vi "Script.vi"(7 "_Rescript in":refnum<class "_Rescript.lvclass">, 8 "error in":errorcluster) -> (0 "error out":errorcluster, 5 "_Rescript out":refnum<class "_Rescript.lvclass">)   [LabVIEW 2025, in "_Rescript.lvlib" / "Msg.lvlib"]
uses:
  Msg.lvlib
  _Rescript/_Rescript.lvclass
  _Shared/Name Specs/Name Specs.lvclass
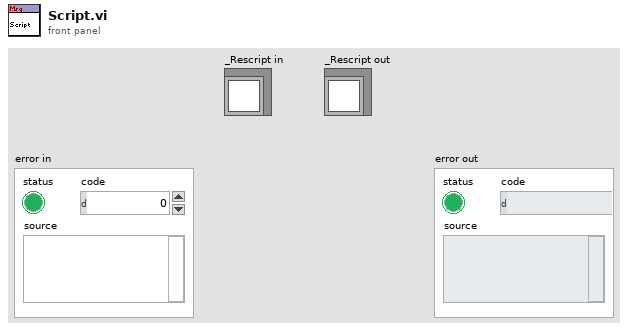
[diagram p1: front panel]
types:
  T1 = typedef "_Shared.lvlib/Name Stuff.ctl" = cluster{"Type (Enum)":T2, "Type (String)":string, "Name Library File Path":path, "Name":string, "Name Type":string}
  T2 = typedef "_Shared.lvlib/Type.ctl" = enum16{"Actor", "Msg"}
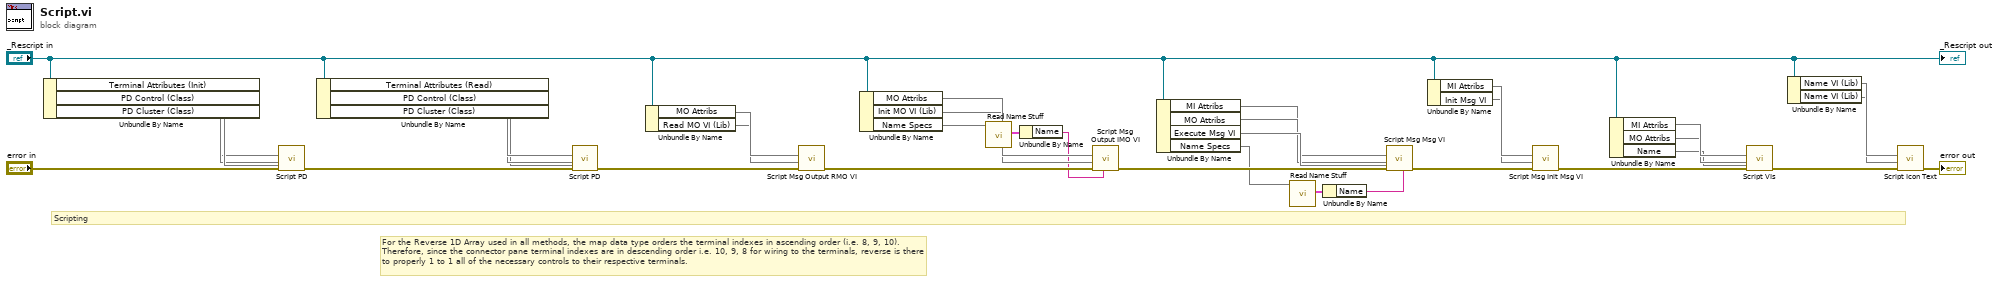
[diagram p0: block diagram]
diagram:
  # "Scripting"
  # "For the Reverse 1D Array used in all methods, the map data type orders the terminal indexes in ascending order (i.e. 8, 9, 10). Therefore, since the connector pane terminal indexes are in descending order i.e. 10, 9, 8 for wiring to the terminals, reverse is there to properly 1 to 1 all of the necessary controls to their respective terminals."
  n1 = Unbundle By Name("_Rescript in") -> ("Terminal Attributes (Init)"=w4, "PD Control (Class)"=w5, "PD Cluster (Class)"=w6)
  n2 = call "Script PD.vi"("PD Cluster"=w6, "error in"="error in", "PD Control"=w5, "Terminal Attributes"=w4) -> ("error out"=w8:errorcluster)  [unwired: 7 in]
  n3 = Unbundle By Name("_Rescript in") -> ("Terminal Attributes (Read)"=w29, "PD Control (Class)"=w28, "PD Cluster (Class)"=w27)
  n4 = call "Script PD.vi"("PD Cluster"=w27, "error in"=w8, "PD Control"=w28, "Terminal Attributes"=w29) -> ("error out"=w7:errorcluster)  [unwired: 7 in]
  n5 = Unbundle By Name("_Rescript in") -> ("MO Attribs"=w23, "Read MO VI (Lib)"=w22)
  n6 = call "Script Msg Output RMO VI.vi"("error in"=w7, "Name Msg Output Refs.Read Msg Output VI"=w22, "Terminal Attributes (Read Msg Output)"=w23) -> ("error out"=w25:errorcluster)  [unwired: 8 in]
  n7 = Unbundle By Name("_Rescript in") -> ("MO Attribs"=w21, "Init MO VI (Lib)"=w20, "Name Specs"=w18)
  n8 = call "Read Name Stuff.vi"("Name Specs in"=w18) -> ("Name Stuff"=w19:T1)  [unwired: 10 in]
  n9 = Unbundle By Name(w19) -> ("Name"=w17:string)
  n10 = call "Script Msg Output IMO VI.vi"("Name"=w17, "error in"=w25, "Name Msg Output Refs.Init Msg Output VI"=w20, "Terminal Attributes (Init Msg Output)"=w21) -> ("error out"=w24:errorcluster)  [unwired: 7 in]
  n11 = Unbundle By Name("_Rescript in") -> ("MI Attribs"=w11, "MO Attribs"=w12, "Execute Msg VI"=w14, "Name Specs"=w15)
  n12 = call "Read Name Stuff.vi"("Name Specs in"=w15) -> ("Name Stuff"=w16:T1)  [unwired: 10 in]
  n13 = Unbundle By Name(w16) -> ("Name"=w13:string)
  n14 = call "Script Msg Msg VI.vi"("Name"=w13, "Name Msg Refs.Msg VI"=w14, "error in"=w24, "Terminal Attributes (Init Msg Output)"=w12, "Terminal Attributes (Read Msg Input)"=w11) -> ("error out"=w33:errorcluster)  [unwired: 6 in]
  n15 = Unbundle By Name("_Rescript in") -> ("MI Attribs"=w10, "Init Msg VI"=w9)
  n16 = call "Script Msg Init Msg VI.vi"("error in"=w33, "Name Msg Refs.Init Msg VI"=w9, "Init Term Attributes (MI)"=w10) -> ("error out"=w26:errorcluster)  [unwired: 8 in]
  n17 = Unbundle By Name("_Rescript in") -> ("MI Attribs"=w32, "MO Attribs"=w31, "Name"=w30)
  n18 = call "Script VIs.vi"("VI Refs"=w30, "error in"=w26, "Terminal Attributes (Read Msg Output)"=w31, "Terminal Attributes (Init Msg Input)"=w32) -> ("error out"=w34:errorcluster)  [unwired: 7 in]
  n19 = Unbundle By Name("_Rescript in") -> ("Name VI (Lib)"=w36, "Name VI (Lib)"=w35)
  n20 = call "Script Icon Text.vi"("error in"=w34, "VI Refs.Name VI"=w35, "Name Refs.Name VI"=w36) -> ("error out"=→"error out":errorcluster)  [unwired: 8 in]
  "_Rescript out" <- "_Rescript in"
